vi "String2Matrix.vi"(1 "Header":string[](array[string]), 2 "R_message 1":string) -> (0 "Array 3":sgl[][](array[numeric]))   [LabVIEW 2022 SP3]
panel:
  out "size(s)":i32[](array[numeric])
  out "Array":sgl[](array[numeric])
  out "subarray":u8[](array[numeric]) format="%x"
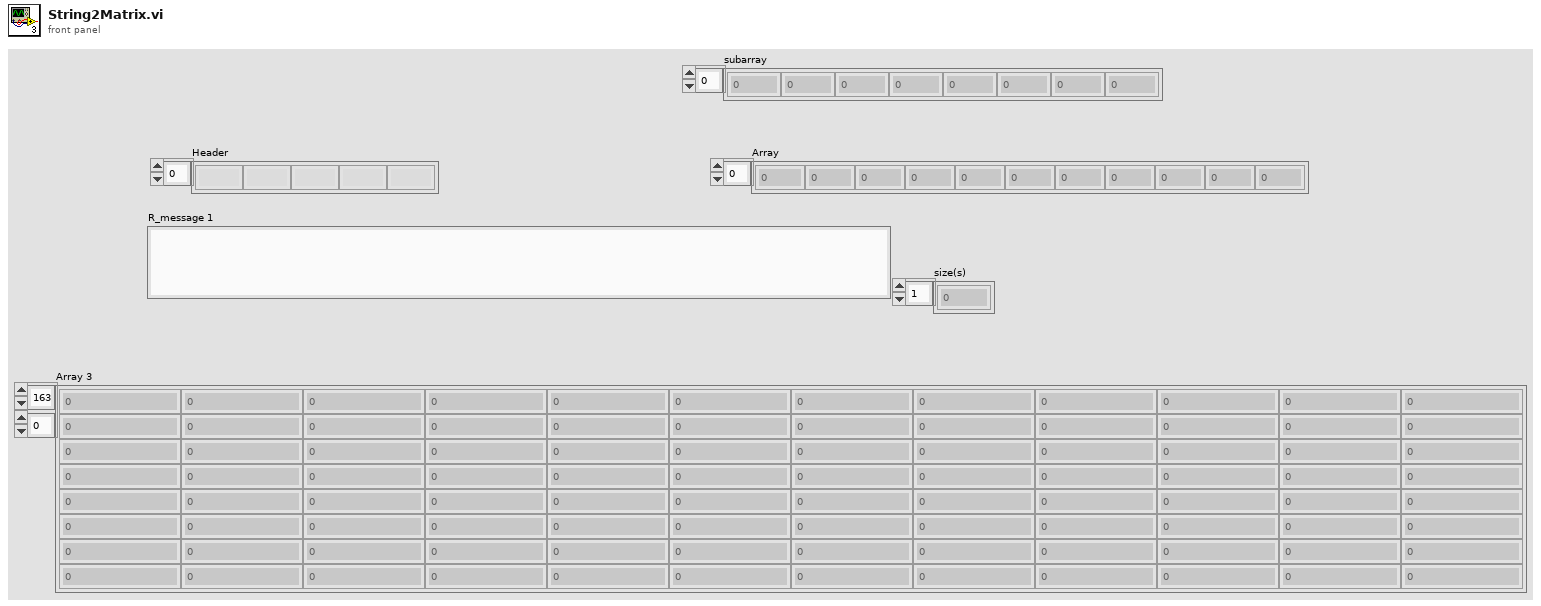
[diagram p1: front panel]
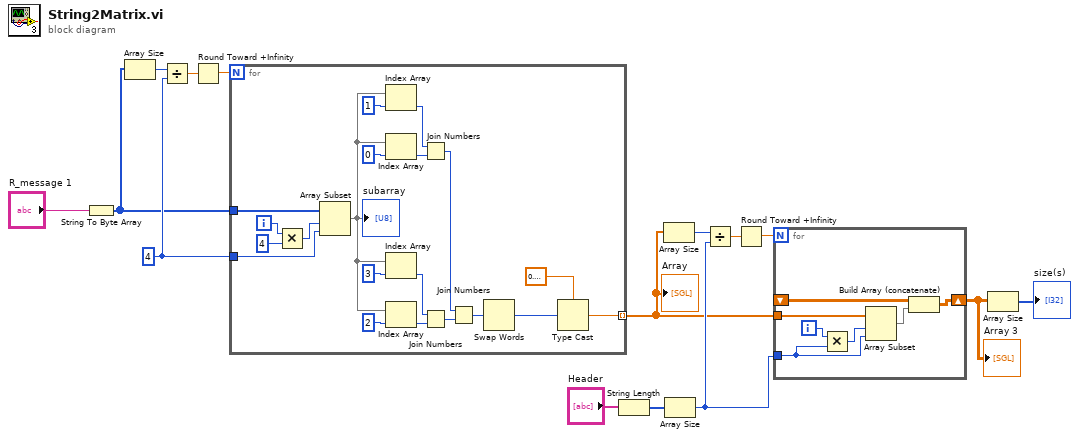
[diagram p0: block diagram]
diagram:
  w11 = 4 ("length")
  n1 = String To Byte Array(string="R_message 1") -> (unsigned byte array=w3:u8[])
  n2 = Array Size(array=w3) -> (size(s)=w12:i32)
  n3 = Divide(x=w12, y=w11) -> (x/y=w10:dbl)
  n4 = Round Toward +Infinity(x=w10) -> (ceil(x): smallest int >= x=w9:dbl)
  n5 = for {
    N: w9 -> [_]
    tunnel: w3 -> [w35]
    tunnel: w11 -> [w34]
    tunnel: [w32] -> w2 mode=indexing
    i -> [w18]
    n6 = Multiply(x=w18, y=4) -> (x*y=w16:i32)
    n7 = Array Subset(array=w35, index=w16, length=w34) -> (w23:u8[])
    "subarray" <- w23
    n8 = Index Array(array=w23, index=1) -> (element=w25:u8)
    n9 = Index Array(array=w23, index=0) -> (element=w24:u8)
    n10 = Index Array(array=w23, index=3) -> (element=w22:u8)
    n11 = Index Array(array=w23, index=2) -> (element=w21:u8)
    n12 = Join Numbers(hi=w25, lo=w24) -> ((hi.lo)=w26:u16)
    n13 = Join Numbers(hi=w22, lo=w21) -> ((hi.lo)=w27:u16)
    n14 = Join Numbers(hi=w26, lo=w27) -> ((hi.lo)=w20:u32)
    n15 = Swap Words(1:w20) -> (0:w19:u32)
    n16 = Type Cast(type=sgl 0.1, x=w19) -> (*(type *) &x=w32:sgl)
  }
  "Array" <- w2
  n17 = String Length(string="Header") -> (length=w14:i32[])
  n18 = Array Size(array=w2) -> (size(s)=w1:i32)
  n19 = Array Size(array=w14) -> (size(s)=w8:i32)
  n20 = Divide(x=w1, y=w8) -> (x/y=w15:dbl)
  n21 = Round Toward +Infinity(x=w15) -> (ceil(x): smallest int >= x=w7:dbl)
  n22 = for {
    N: w7 -> [_]
    tunnel: w2 -> [w42]
    tunnel: w8 -> [w36]
    shift-right: [w41] -> w4
    shift-left: _ -> [w39]
    i -> [w38]
    n23 = Multiply(x=w38, y=w36) -> (x*y=w37:i32)
    n24 = Array Subset(array=w42, index=w37, length=w36) -> (w40:sgl[])
    n25 = Build Array (concatenate)(w39, w40) -> (w41:sgl[][])
  }
  "Array 3" <- w4
  n26 = Array Size(array=w4) -> (size(s)=→"size(s)":i32[])
